vi "Connect.vi"(8 "error in":errorcluster, 11 "TC01 in":refnum<class "TC01.lvclass">) -> (0 "error out":errorcluster, 3 "TC01 out":refnum<class "TC01.lvclass">)   [LabVIEW 2018, in "TC01.lvlib" / "TC01.lvclass"]
uses:
  TC01.lvclass
  TC01.lvclass/TC01.ctl
  <vilib>/DAQmx/create/channels.llb/DAQmx Create Channel (AI-Temperature-Thermocouple).vi
  PPLs/Thermocouple/Thermocouple.lvlibp/Thermocouple.lvclass
  C:/Projects/LabVIEW/PPLs/Thermocouple/Thermocouple.lvlibp/Thermocouple.lvclass
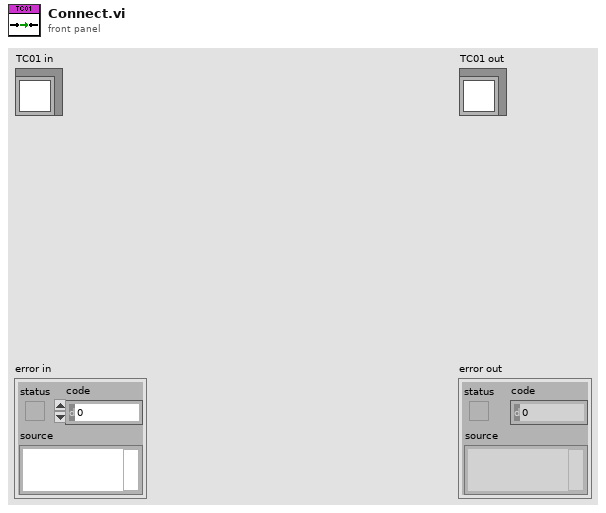
[diagram p1: front panel]
types:
  T1 = typedef "Thermocouple.lvlibp/Thermocouple Type.ctl" = enum16{"J", "K", "N", "R", "S", "T", "B", "E"}
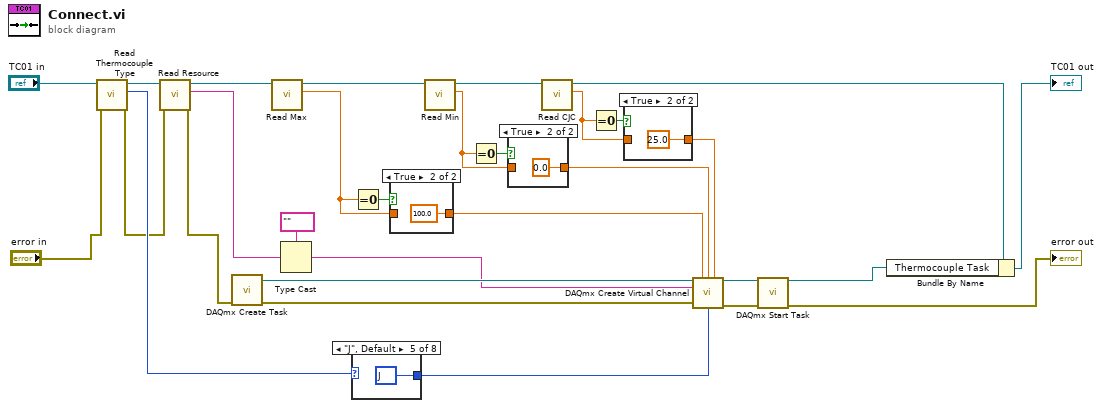
[diagram p0: block diagram]
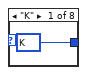
[diagram p5: hidden frame]
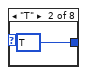
[diagram p6: hidden frame]
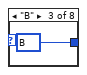
[diagram p7: hidden frame]
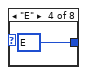
[diagram p8: hidden frame]
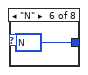
[diagram p9: hidden frame]
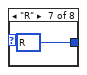
[diagram p10: hidden frame]
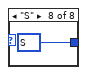
[diagram p11: hidden frame]
diagram:
  n1 = call "Read Thermocouple Type.vi"("error in (no error)"="error in", "Thermocouple in"="TC01 in") -> ("error out"=w18:errorcluster, "Thermocouple Type"=w21:T1, "Thermocouple out"=w19:refnum<class "TC01.lvclass">)  [unwired: 7 in]
  n2 = call "Read Resource.vi"("error in (no error)"=w18, "Thermocouple in"=w19) -> ("error out"=w17:errorcluster, "Resource"=w16:tag, "Thermocouple out"=w13:refnum<class "TC01.lvclass">)  [unwired: 7 in]
  n3 = call <vilib>:"DAQmx Create Task.vi"("error in"=w17) -> ("task out"=w28:refnum<k21>, "error out"=w27:errorcluster)  [unwired: 13 in]
  n4 = call "Read Max.vi"("Thermocouple in"=w13) -> ("Max"=w7:dbl, "Thermocouple out"=w12:refnum<class "TC01.lvclass">)  [unwired: 8 in, 1 out]
  n5 = Type Cast(type=tag "" ("physical channels"), x=w16) -> (*(type *) &x=w14:tag)
  n6 = case shown="\"J\", Default" w21 {
    tunnel: [w31 w32 w33 w34 w35 w36 w37 w38] -> w20
    frame "K" {
      w31 = 10073 items=["J"=10072, "K"=10073, "N"=10077, "R"=10082, "S"=10085, "T"=10086, "B"=10047, "E"=10055] ("thermocouple type")
    }
    frame "T" {
      w32 = 10086 items=["J"=10072, "K"=10073, "N"=10077, "R"=10082, "S"=10085, "T"=10086, "B"=10047, "E"=10055] ("thermocouple type")
    }
    frame "B" {
      w33 = 10047 items=["J"=10072, "K"=10073, "N"=10077, "R"=10082, "S"=10085, "T"=10086, "B"=10047, "E"=10055] ("thermocouple type")
    }
    frame "E" {
      w34 = 10055 items=["J"=10072, "K"=10073, "N"=10077, "R"=10082, "S"=10085, "T"=10086, "B"=10047, "E"=10055] ("thermocouple type")
    }
    frame "J", Default {
      w35 = 10072 items=["J"=10072, "K"=10073, "N"=10077, "R"=10082, "S"=10085, "T"=10086, "B"=10047, "E"=10055] ("thermocouple type")
    }
    frame "N" {
      w36 = 10077 items=["J"=10072, "K"=10073, "N"=10077, "R"=10082, "S"=10085, "T"=10086, "B"=10047, "E"=10055] ("thermocouple type")
    }
    frame "R" {
      w37 = 10082 items=["J"=10072, "K"=10073, "N"=10077, "R"=10082, "S"=10085, "T"=10086, "B"=10047, "E"=10055] ("thermocouple type")
    }
    frame "S" {
      w38 = 10085 items=["J"=10072, "K"=10073, "N"=10077, "R"=10082, "S"=10085, "T"=10086, "B"=10047, "E"=10055] ("thermocouple type")
    }
  }
  n7 = Equal To 0?(x=w7) -> (x = 0?=w8:bool)
  n8 = case shown="True" w8 {
    tunnel: [w39 100.0 ("maximum value")] -> w9
    tunnel: w7 -> [w39 _]
    frame False {
    }
    frame True {
    }
  }
  n9 = call "Read Min.vi"("Thermocouple in"=w12) -> ("Min"=w5:dbl, "Thermocouple out"=w11:refnum<class "TC01.lvclass">)  [unwired: 8 in, 1 out]
  n10 = Equal To 0?(x=w5) -> (x = 0?=w6:bool)
  n11 = case shown="True" w6 {
    tunnel: [w41 0.0] -> w4
    tunnel: w5 -> [w41 _]
    frame False {
    }
    frame True {
    }
  }
  n12 = call "Read CJC.vi"("Thermocouple in"=w11) -> ("CJC"=w2:dbl, "Thermocouple out"=w10:refnum<class "TC01.lvclass">)  [unwired: 8 in, 1 out]
  n13 = Equal To 0?(x=w2) -> (x = 0?=w3:bool)
  n14 = case shown="True" w3 {
    tunnel: w2 -> [w43 _]
    tunnel: [w43 25.0 ("cjc value")] -> w1
    frame False {
    }
    frame True {
    }
  }
  n15 = call-poly <vilib>:"DAQmx Create Virtual Channel.vi"("task in"=w28, "maximum value"=w9, "minimum value"=w4, "physical channels"=w14, "error in"=w27, "thermocouple type"=w20, "cjc value"=w1) -> ("task out"=w25:refnum<k21>, "error out"=w22:errorcluster)  [unwired: 7 in]
  n16 = call <vilib>:"DAQmx Start Task.vi"("task/channels in"=w25, "error in"=w22) -> ("task out"=w24:refnum<k21>, "error out"=→"error out":errorcluster)  [unwired: 12 in]
  n17 = Bundle By Name(cluster=w10, "Thermocouple Task"=w24) -> (→"TC01 out":refnum<class "TC01.lvclass">)
